vi "Update.vi"(8 "error in":errorcluster, 10 "object ref in":T1, 11 "Data Grid in":refnum<class "Data Grid.lvclass">) -> (0 "error out":errorcluster, 2 "object ref out":T1, 3 "Data Grid out":refnum<class "Data Grid.lvclass">)   [LabVIEW 2013, in "Table Manager.lvlib" / "Data Grid.lvclass"]
uses:
  Data Grid.lvclass
  Table Manager/object ref.ctl
  <vilib>/NI/DCAF/Tag Editor Core/Configuration Editor/Classes/Engine Parent/Engine Parent Editor Node.lvclass
  <vilib>/NI/DCAF/Tag Editor Core/Configuration Editor/Classes/Module editor node/module editor node.lvclass
  Data Grid.lvclass/Data Grid.ctl
  Table Manager/Table Manager.lvclass
  <vilib>/DataGrid for LabVIEW/source/DataGridView/DataGridView.lvclass
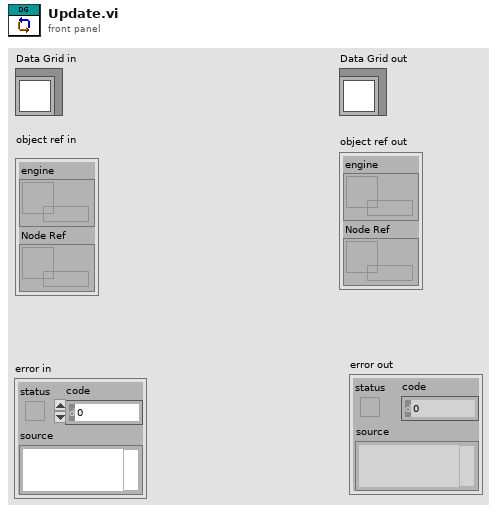
[diagram p1: front panel]
types:
  T1 = typedef "Table Manager.lvlib/Table Manager.lvclass/object ref.ctl" = cluster{"engine":refnum<data-value>, "Node Ref":refnum<data-value>}
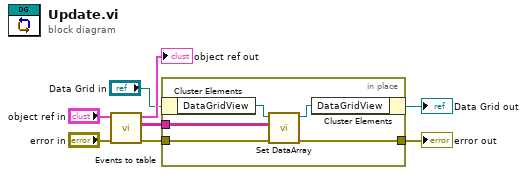
[diagram p0: block diagram]
diagram:
  n1 = call "Events to table.vi"("error in (no error)"="error in", "object ref in"="object ref in") -> ("error out"=w1:errorcluster, "table"=w5:string[][], "object ref out"=→"object ref out":T1)  [unwired: 7 in]
  n2 = in-place {
    in-place-border: w5 -> [w11]
    in-place-border: [w10] -> w3
    in-place-border: w1 -> [w9]
    n3 = in-place-cluster #1("Data Grid in") -> ("DataGridView"=w13:refnum<class "DataGridView.lvclass">)
    n4 = call <vilib>:"Set DataArray.vi"("error in"=w9, "Data"=w11, "DataGridView in"=w13) -> ("error out"=w10:errorcluster, "DataGridView out"=w12:refnum<class "DataGridView.lvclass">)  [unwired: 7 in]
    n5 = in-place-cluster #1("DataGridView"=w12) -> (→"Data Grid out":refnum<class "Data Grid.lvclass">)
  }
  "error out" <- w3
